vi "Check position str.vi"(7 "mm/step":dbl=0.0025 format="%#_13g", 8 "error in (no error)":errorcluster, 9 "Motor params":T1={"Tipo"=2, "Dirección"=1, "N°. Pasos"=1, "Frecuencia (Hz)"=100, "Tipo de paso"=100} {"Tipo de paso" items=["", "Medio paso", "Paso completo"]; "Dirección" items=["", "Izquierda", "Derecha"]; "Tipo" items=["", "Unipolar", "Bipolar"]}, 10 "Position in":dbl, 11 "String read":string) -> (0 "error out":errorcluster, 2 "End?":bool, 3 "Position out":dbl)   [LabVIEW 2020, in "Control de MaP.lvlib"]
doc: "Converts the read string into a double and updates the Position of the motor. If the read string is 'fin', it keeps the last position and returns the End flag as True."
uses:
  Control de MaP.lvlib
  Controls/Command to motor.ctl
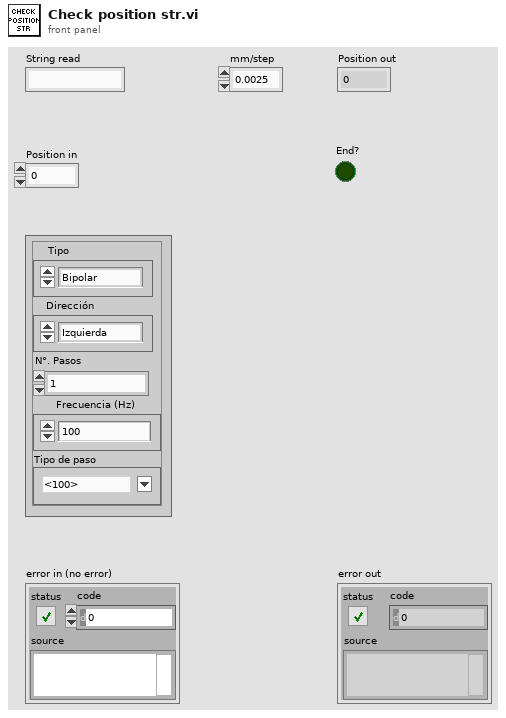
[diagram p1: front panel]
types:
  T1 = typedef "Control de MaP.lvlib/Command to motor.ctl" = cluster{"Tipo":u8, "Dirección":u8, "N°. Pasos":u16, "Frecuencia (Hz)":u8, "Tipo de paso":u8}
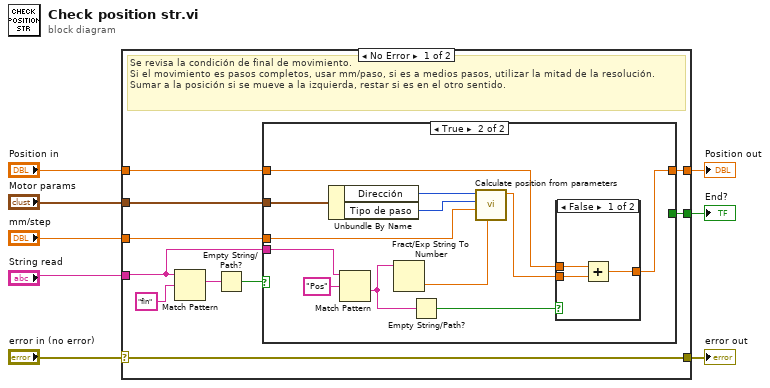
[diagram p0: block diagram]
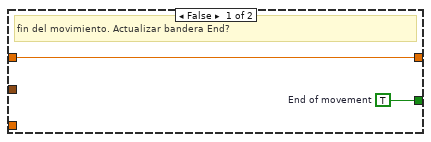
[diagram p2: hidden frame]
diagram:
  n1 = case shown="No Error" "error in (no error)" {
    selector: "error in (no error)" -> [w18 w38]
    tunnel: [w17 w37] -> w8
    tunnel: "Position in" -> [w16 w37]
    tunnel: "String read" -> [w9 _]
    tunnel: [w18 w38] -> w4
    tunnel: "Motor params" -> [w15 _]
    tunnel: "mm/step" -> [w14 _]
    tunnel: [w10 _] -> w1
    frame No Error {
      # "Se revisa la condición de final de movimiento.\nSi el movimiento es pasos completos, usar mm/paso, si es a medios pasos, utilizar la mitad de la resolución. Sumar a la posición si se mueve a la izquierda, restar si es en el otro sentido."
      n2 = Match Pattern(string=w9, regular expression="fin") -> (match substring=w12:string)  [unwired: 1 in, 3 out]
      n3 = Empty String/Path?(string/path=w12) -> (empty?=w11:bool)
      n4 = case shown="True" w11 {
        tunnel: [w20 w29] -> w17
        tunnel: w16 -> [w20 w28]
        tunnel: w15 -> [_ w26]
        tunnel: w14 -> [_ w25]
        tunnel: [w19 _] -> w10
        tunnel: w9 -> [_ w21]
        frame False {
          w19 = TRUE  # End of movement
          # "fin del movimiento. Actualizar bandera End?"
        }
        frame True {
          n5 = Unbundle By Name(w26) -> ("Dirección"=w30:u8, "Tipo de paso"=w31:u8)
          n6 = Match Pattern(string=w21, regular expression="Pos") -> (after substring=w23:string)  [unwired: 1 in, 3 out]
          n7 = Fract/Exp String To Number(string=w23) -> (number=w24:dbl)  [unwired: 3 in, 1 out]
          n8 = Empty String/Path?(string/path=w23) -> (empty?=w27:bool)
          n9 = call "Calculate position from parameters.vi"("Current step"=w24, "mm/step"=w25, "Tipo de paso"=w31, "Motor direction"=w30) -> ("Position adjustment"=w22:dbl)  [unwired: 6 in, 1 out]
          n10 = case shown="False" w27 {
            tunnel: [w35 w36] -> w29
            tunnel: w28 -> [w34 w36]
            tunnel: w22 -> [w33 _]
            frame False {
              n11 = Add(x=w34, y=w33) -> (x+y=w35:dbl)
            }
            frame True {
            }
          }
        }
      }
    }
    frame Error {
    }
  }
  "Position out" <- w8
  "error out" <- w4
  "End?" <- w1
